vi "Bias2_load.vi"() -> ()   [LabVIEW 2022 SP3]
panel:
  out "size(s)":i32
  out "Init Data Out":sgl[](array[numeric])
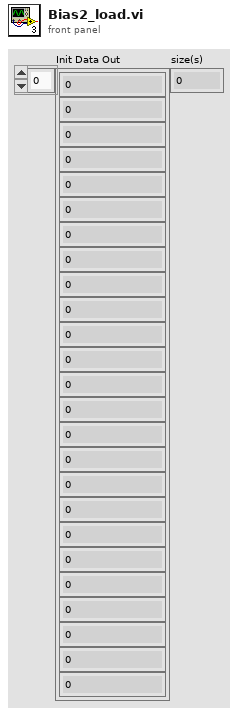
[diagram p1: front panel]
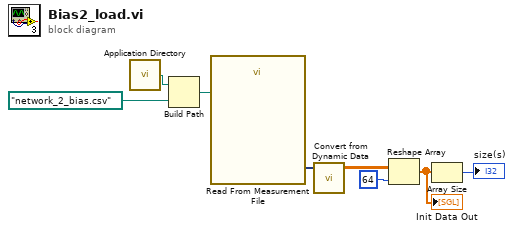
[diagram p0: block diagram]
diagram:
  n1 = call <vilib>:"Application Directory.vi"() -> ("Application Directory"=w7:path)
  n2 = Build Path(base path=w7, name or relative path=path "network_2_bias.csv" ("default name")) -> (appended path=w5:path)
  n3 = call "Read From Measurement File"("Filename"=w5) -> ("Signals"=w4:dynamicdata)  [unwired: 5 in, 5 out]
  n4 = call "Convert from Dynamic Data"("Dynamic Data Type"=w4) -> ("Array"=w3:dbl[][])  [unwired: 3 in]
  n5 = Reshape Array(w3, 64 ("dimension size")) -> (w1:dbl[])
  "Init Data Out" <- w1
  n6 = Array Size(array=w1) -> (size(s)=→"size(s)":i32)
